vi "ROI坐标转换.vi"() -> ()   [LabVIEW 2018]
panel:
  out "Image":T1(plugin-control)
  in  "路径":path
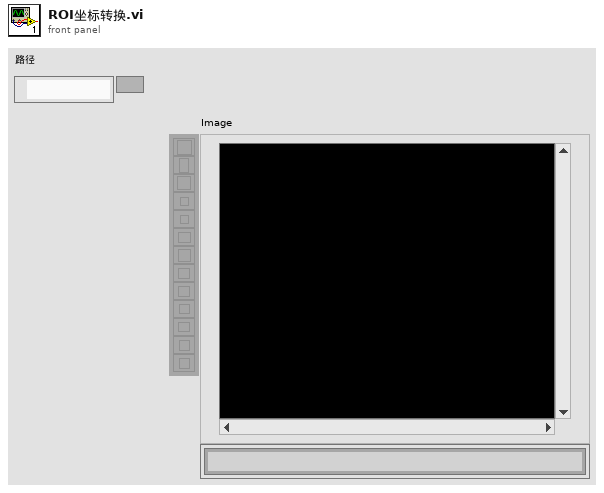
[diagram p1: front panel]
types:
  T1 = typedef "IMAQ Image.ctl" = refnum<image>
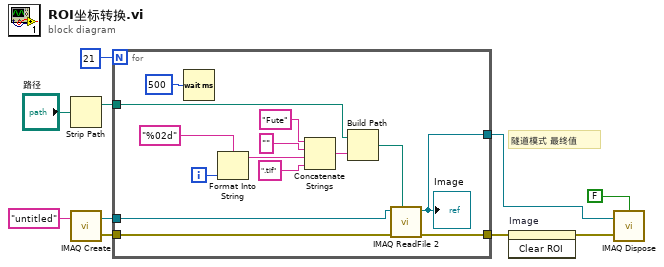
[diagram p0: block diagram]
diagram:
  # "隧道模式 最终值"
  n1 = Strip Path(path="路径") -> (stripped path=w8:path)  [unwired: 1 out]
  n2 = call "IMAQ Create"("Image Name"="untitled") -> ("New Image"=w7:T1, "error out"=w6:errorcluster)  [unwired: 4 in]
  n3 = for {
    N: 21 -> [_]
    tunnel: w8 -> [w15]
    tunnel: w7 -> [w24]
    tunnel: w6 -> [w23]
    tunnel: [w13] -> w4
    tunnel: [w12] -> w2
    i -> [w22]
    n4 = Wait (ms)(milliseconds to wait=u32 500 ("等待时间（毫秒）")) -> ()  [unwired: 1 out]
    n5 = Format Into String(format string="%02d" ("格式字符串"), w22) -> (resulting string=w20:string)  [unwired: 2 in, 1 out]
    n6 = Concatenate Strings("Fute" ("字符串"), "" ("字符串"), w20, ".tif" ("字符串")) -> (w16:string)
    n7 = Build Path(base path=w15, name or relative path=w16) -> (appended path=w14:path)
    n8 = call "IMAQ ReadFile 2"("File Path"=w14, "error in (no error)"=w23, "Image"=w24) -> ("error out"=w13:errorcluster, "Image Out"=w12:T1)  [unwired: 4 in, 3 out]
    "Image" <- w12
  }
  n9 = invoke on="Image" class="ImageControl" method="Clear ROI"(error in=w4) -> (error out=w3:errorcluster)  [unwired: 2 in, 2 out]
  n10 = call "IMAQ Dispose"("All Images? (No)"=FALSE, "Image"=w2, "error in (no error)"=w3) -> ()  [unwired: 3 in, 1 out]
